vi "QueryServer_Event_Close.vi"(0 "gRPCid":T1, 3 "error in (no error)":errorcluster) -> (10 "error out":errorcluster)   [LabVIEW 2019, in "labview-grpc-query-server.lvlib"]
uses:
  labview-grpc-query-server.lvlib
  QueryServer_gRPCid.ctl
  build/Debug/labview_measurement_server.dll
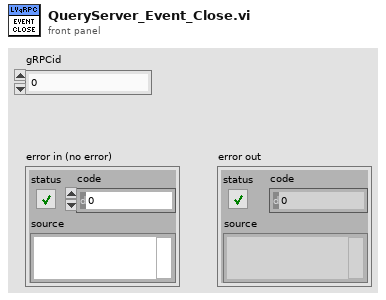
[diagram p1: front panel]
types:
  T1 = typedef "labview-grpc-query-server.lvlib/QueryServer_gRPCid.ctl" = u64
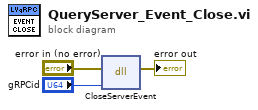
[diagram p0: block diagram]
diagram:
  n1 = dll-call lib="C:/dev/labview-grpc-measurement-server/build/Debug/labview_measurement_server.dll" fn="CloseServerEvent"(error in="error in (no error)", "id"="gRPCid") -> (error out=→"error out":errorcluster)  [unwired: 4 in, 1 out]
